vi "Build Pre-Filter Rejection.vi"(7 "Virtual Memory Unit in":refnum<class "Virtual Memory Unit.lvclass">, 8 "error in (no error)":errorcluster, 11 "Bus Monitor in":refnum<class "Bus Monitor.lvclass">) -> (0 "error out":errorcluster, 3 "Bus Monitor out":refnum<class "Bus Monitor.lvclass">, 5 "Virtual Memory Unit out":refnum<class "Virtual Memory Unit.lvclass">)   [LabVIEW 2020, in "BCI-1553 API.lvlib" / "Bus Monitor.lvclass"]
doc: "Force every monitorable RT & subaddress to be unmonitored by default. The addition of filters will set these various RT and subaddresses to be monitored by the bus monitor."
uses:
  Bus Monitor.lvclass
  Dependencies/Virtual Memory Unit/Virtual Memory Unit.lvclass
  Bus Monitor.lvclass/Bus Monitor.ctl
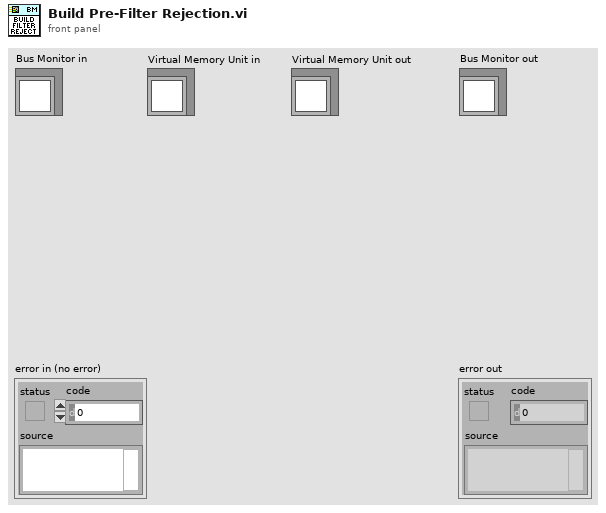
[diagram p1: front panel]
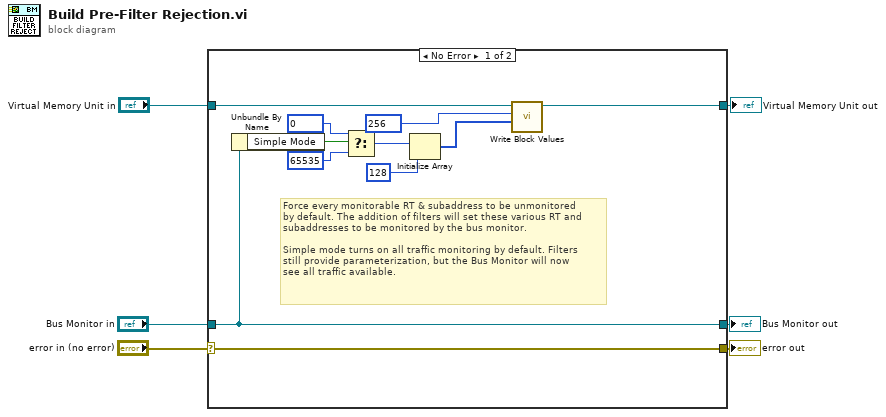
[diagram p0: block diagram]
diagram:
  n1 = case shown="No Error" "error in (no error)" {
    selector: "error in (no error)" -> [w17 w20]
    tunnel: [w17 w20] -> w5
    tunnel: [w11 w19] -> w3
    tunnel: "Bus Monitor in" -> [w11 w19]
    tunnel: [w14 w18] -> w2
    tunnel: "Virtual Memory Unit in" -> [w15 w18]
    frame No Error {
      # "Force every monitorable RT & subaddress to be unmonitored\nby default. The addition of filters will set these various RT and\nsubaddresses to be monitored by the bus monitor.\n\nSimple mode turns on all traffic monitoring by default. Filters\nstill provide parameterization, but the Bus Monitor will now \nsee all traffic available."
      n2 = Unbundle By Name(w11) -> ("Simple Mode"=w10:bool)
      n3 = Select(t=u16 0, s=w10, f=u16 65535) -> (s? t:f=w8:u16)
      n4 = Initialize Array(w8, 128) -> (w13:u16[])
      n5 = call "Write Block Values.vi"("Write Block"=w13, "Start Index"=256, "Virtual Memory Unit in"=w15) -> ("Virtual Memory Unit out"=w14:refnum<class "Virtual Memory Unit.lvclass">)  [unwired: 7 in, 1 out]
    }
    frame Error {
    }
  }
  "error out" <- w5
  "Bus Monitor out" <- w3
  "Virtual Memory Unit out" <- w2
